vi "IL Sample in Container.vi"(4 "Add to (Deny)":T2, 5 "Ignore (F)":bool, 6 "Condition Samples":refnum<class "Sample.lvclass">[](array[class]), 7 "Stop Self on IL? (T)":bool=TRUE, 8 "error in (no error)":errorcluster, 10 "Sample Container":T1, 11 "Interlock Chain in":refnum<class "Interlock Chain.lvclass">) -> (0 "error out":errorcluster, 2 "IL Sample in Container":refnum<class "Interlock.lvclass">, 3 "Interlock Chain out":refnum<class "Interlock Chain.lvclass">)   [LabVIEW 2015, in "cRIO-Carbondioxide.lvlib" / "cRIO-CO2.lvlib" / "cRIO-CO2.lvclass"]
uses:
  cRIO-CO2.lvclass
  Interlocks/Interlock Chain/Interlock Chain.lvclass
  Interlocks/Controls/Add IL to -Enumerator.ctl
  Interlocks/Interlock/Interlock.lvclass
  subs/Sample/Sample.lvclass
  Controls/Sample Container.ctl
  Interlocks/Interlock Sample/Interlock Sample.lvclass
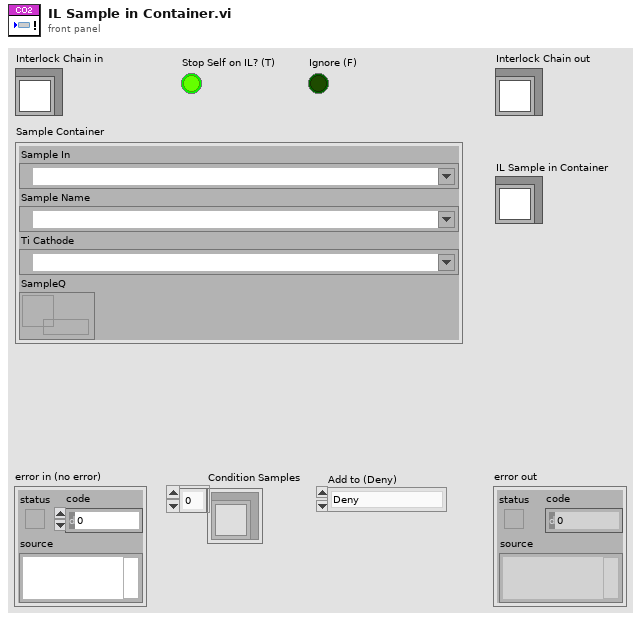
[diagram p1: front panel]
types:
  T1 = typedef "Sample Container.ctl" = cluster{"Sample In":refnum<k21>, "Sample Name":refnum<k21>, "Ti Cathode":refnum<k21>, "SampleQ":refnum<queue>}
  T2 = typedef "Add IL to -Enumerator.ctl" = enum16{"Deny", "Allow", "None"}
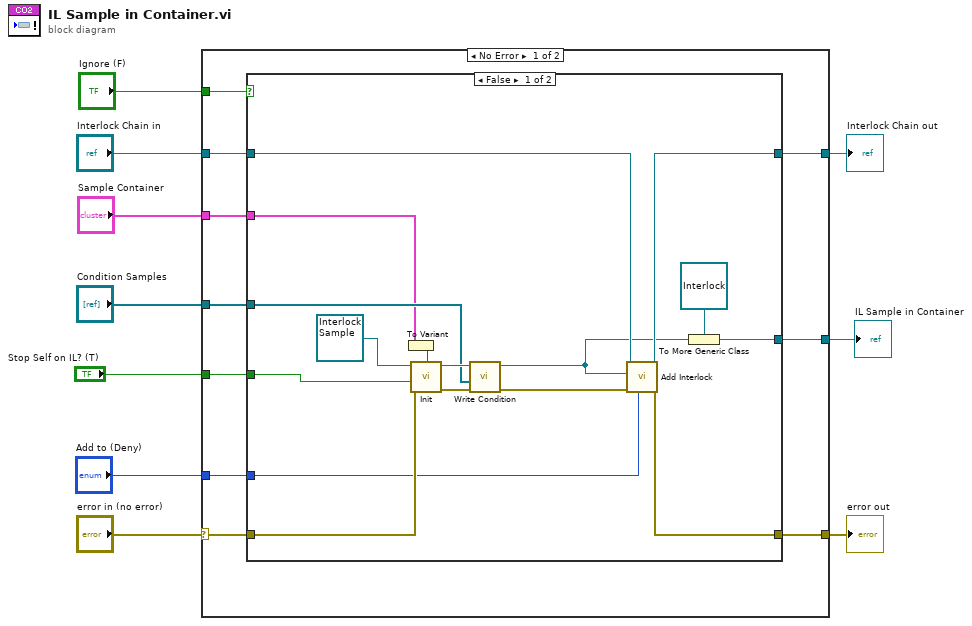
[diagram p0: block diagram]
diagram:
  n1 = case shown="No Error" "error in (no error)" {
    selector: "error in (no error)" -> [w17 w40]
    tunnel: [w16 w40] -> w9
    tunnel: [w18 w39] -> w7
    tunnel: "Interlock Chain in" -> [w19 w39]
    tunnel: "Condition Samples" -> [w20 _]
    tunnel: "Add to (Deny)" -> [w15 _]
    tunnel: [w14 _] -> w5
    tunnel: "Stop Self on IL? (T)" -> [w13 _]
    tunnel: "Ignore (F)" -> [w12 _]
    tunnel: "Sample Container" -> [w11 _]
    frame No Error {
      n2 = case shown="False" w12 {
        tunnel: w20 -> [w24 _]
        tunnel: w19 -> [w33 w38]
        tunnel: [w32 w38] -> w18
        tunnel: w17 -> [w31 w37]
        tunnel: [w30 w37] -> w16
        tunnel: w15 -> [w29 _]
        tunnel: [w28 _] -> w14
        tunnel: w13 -> [w25 _]
        tunnel: w11 -> [w23 _]
        frame False {
          n3 = To Variant(anything=w23) -> (Variant=w26:variant)
          n4 = call-dynamic "Init.vi"("Sample Containers SHV (Array!)"=w26, "error in (no error)"=w31, "Stop Self on IL? (T)"=w25, "Interlock Sample in"=refnum<class "Interlock Sample.lvclass"> refnum ("Interlock Bool.lvclass")) -> ("error out"=w34:errorcluster, "Interlock Sample out"=w35:refnum<class "Interlock Sample.lvclass">)  [unwired: 6 in]
          n5 = call "Write Condition.vi"("error in (no error)"=w34, "Samples"=w24, "Interlock Sample in"=w35) -> ("error out"=w22:errorcluster, "Interlock Sample out"=w21:refnum<class "Interlock Sample.lvclass">)  [unwired: 7 in]
          n6 = call "Add Interlock.vi"("Add to (Deny)"=w29, "error in (no error)"=w22, "Interlock.lvclass"=w21, "Interlock Chain in"=w33) -> ("error out"=w30:errorcluster, "Interlock Chain out"=w32:refnum<class "Interlock Chain.lvclass">)  [unwired: 6 in]
          n7 = To More Generic Class(target class=refnum<class "Interlock.lvclass"> refnum ("Interlock.lvclass"), reference=w21) -> (generic class reference=w28:refnum<class "Interlock.lvclass">)
        }
        frame True {
        }
      }
    }
    frame Error {
    }
  }
  "error out" <- w9
  "Interlock Chain out" <- w7
  "IL Sample in Container" <- w5
